vi "ble_discover_stop.vi"(8 "error in (no error)":errorcluster, 11 "COM Bluegiga in":refnum<visa-resource-name>) -> (0 "error out":errorcluster, 1 "payload":u8[](array[numeric]), 2 "success?":bool, 3 "COM Bluegiga out":refnum<visa-resource-name>)   [LabVIEW 2013]
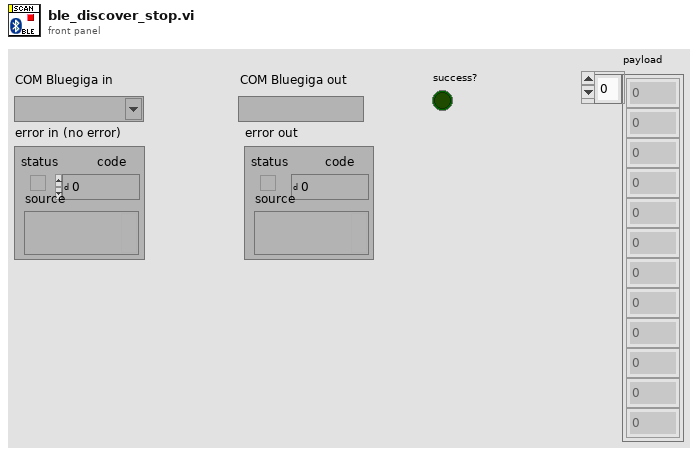
[diagram p1: front panel]
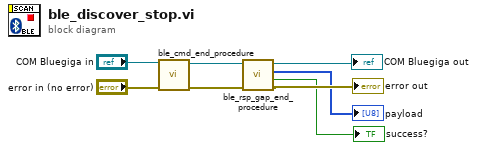
[diagram p0: block diagram]
diagram:
  n1 = call "ble_cmd_end_procedure.vi"("error in (no error)"="error in (no error)", "COM Bluegiga in"="COM Bluegiga in") -> ("error out"=w5:errorcluster, "COM Bluegiga out"=w6:refnum<visa-resource-name>)  [unwired: 8 in]
  n2 = call "ble_rsp_gap_end_procedure.vi"("error in (no error)"=w5, "COM Bluegiga in"=w6) -> ("error out"=→"error out":errorcluster, "success?"=→"success?":bool, "full message package"=→"payload":u8[], "COM Bluegiga out"=→"COM Bluegiga out":refnum<visa-resource-name>)  [unwired: 6 in]
